vi "Parse Structures.vi"(8 "error in":errorcluster, 11 "ParseGDSII in":refnum<class "ParseGDSII.lvclass">) -> (0 "error out":errorcluster, 2 "Geometric":refnum<class "Geometric.lvclass">[](array[class]), 3 "ParseGDSII out":refnum<class "ParseGDSII.lvclass">)   [LabVIEW 2019, in "ParseGDSII.lvclass"]
uses:
  ParseGDSII.lvclass
  Elements/Geometric.lvclass
  ParseGDSII.lvclass/ParseGDSII.ctl
  Tree/Tree.lvclass
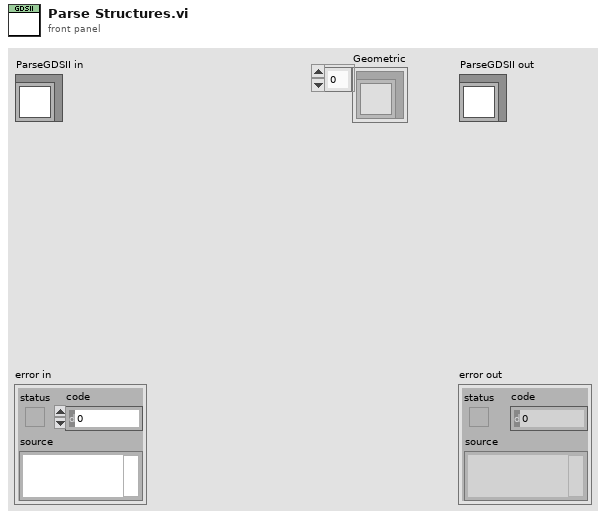
[diagram p1: front panel]
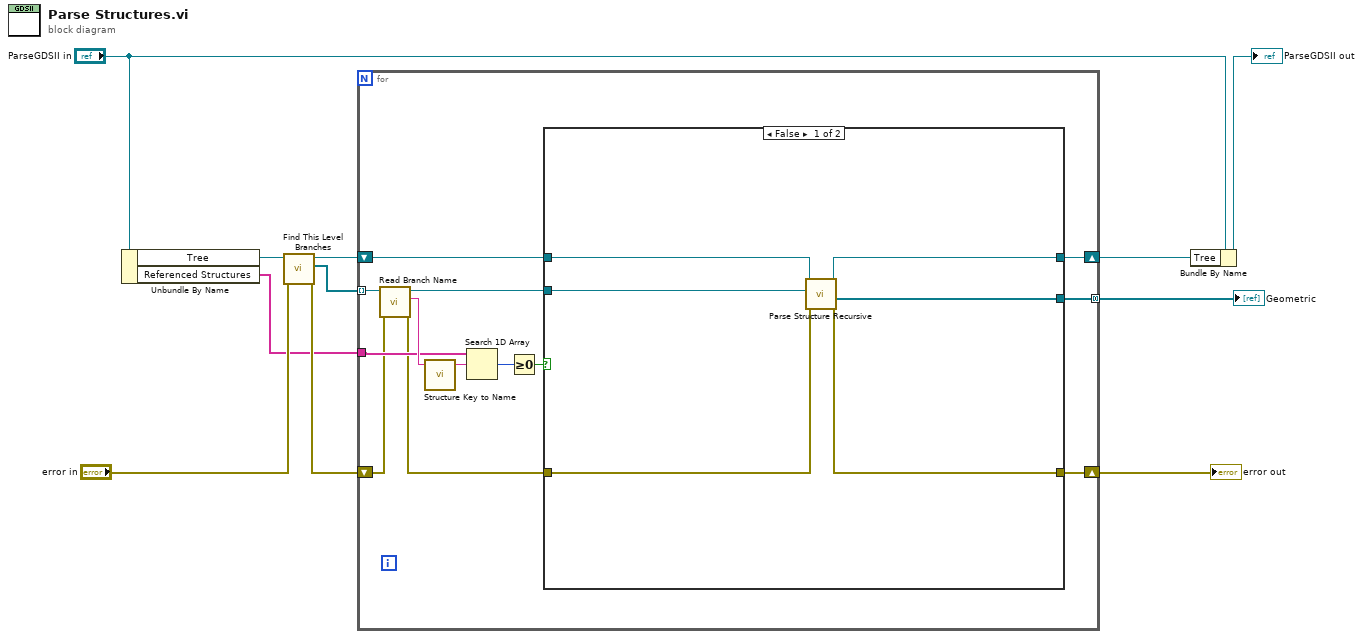
[diagram p0: block diagram]
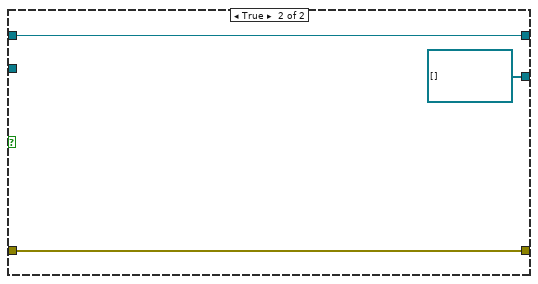
[diagram p2: hidden frame]
diagram:
  n1 = Unbundle By Name("ParseGDSII in") -> ("Tree"=w10:refnum<class "Tree.lvclass">, "Referenced Structures"=w2:string[])
  n2 = call "Find This Level Branches.vi"("error in"="error in", "Tree in"=w10) -> ("error out"=w5:errorcluster, "Branches"=w8:refnum<class "Tree.lvclass">[], "Tree out"=w9:refnum<class "Tree.lvclass">)  [unwired: 7 in]
  n3 = for {
    shift-right: [w17] -> w4
    shift-left: w9 -> [w18]
    tunnel: w8 -> [w13] mode=indexing
    shift-right: [w15] -> w6
    shift-left: w5 -> [w19]
    tunnel: w2 -> [w20]
    tunnel: [w12] -> w1 mode=concatenating
    n4 = call "Read Branch Name.vi"("error in"=w19, "Tree in"=w13) -> ("error out"=w16:errorcluster, "Branch Name"=w24:string, "Tree out"=w14:refnum<class "Tree.lvclass">)  [unwired: 7 in]
    n5 = call "Structure Key to Name.vi"("Key"=w24) -> ("Name"=w23:string)  [unwired: 4 in]
    n6 = Search 1D Array(1D array=w20, element=w23) -> (index of element=w22:i32)  [unwired: 1 in]
    n7 = Greater Or Equal To 0?(x=w22) -> (x >= 0?=w21:bool)
    n8 = case shown="False" w21 {
      tunnel: w18 -> [w29 w33]
      tunnel: w14 -> [w28 _]
      tunnel: [w30 w33] -> w17
      tunnel: w16 -> [w27 w32]
      tunnel: [w26 w32] -> w15
      tunnel: [w25 refnum<class "Geometric.lvclass">[] [] ("Geometric")] -> w12
      frame False {
        n9 = call "Parse Structure Recursive.vi"("error in"=w27, "Structure In"=w28, "Tree In"=w29) -> ("error out"=w26:errorcluster, "Geometric"=w25:refnum<class "Geometric.lvclass">[], "Tree Out"=w30:refnum<class "Tree.lvclass">)  [unwired: 5 in, 1 out]
      }
      frame True {
      }
    }
  }
  "error out" <- w6
  "Geometric" <- w1
  n10 = Bundle By Name(cluster="ParseGDSII in", "Tree"=w4) -> (→"ParseGDSII out":refnum<class "ParseGDSII.lvclass">)
